vi "Test HP3488A.vi"() -> ()   [LabVIEW 2015]
panel:
  in  "Card Number":u8=1 min=1 max=5 step=1
  in  "VISA resource name":refnum<visa-resource-name>
  in  "stop":bool
  in  "Channel to select":T1(ring)
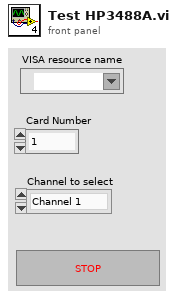
[diagram p1: front panel]
types:
  T1 = enum16{"Channel 1", "Channel 2", "Channel 3", "Channel 4"}
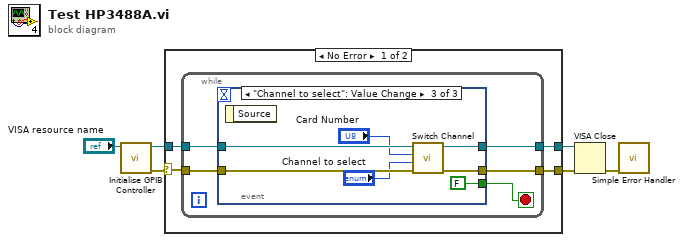
[diagram p0: block diagram]
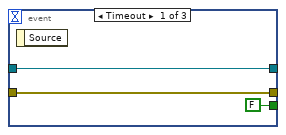
[diagram p2: hidden frame]
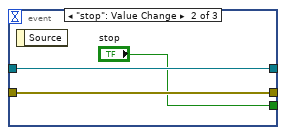
[diagram p3: hidden frame]
diagram:
  n1 = call "Initialise GPIB Controller.vi"("VISA resource name"="VISA resource name") -> ("error out"=w2:errorcluster, "VISA resource name out"=w6:refnum<visa-resource-name>)  [unwired: 5 in]
  n2 = case shown="No Error" w2 {
    selector: w2 -> [w7 w29]
    tunnel: w6 -> [w10 w30]
    tunnel: [w9 w30] -> w5
    tunnel: [w8 w29] -> w4
    frame No Error {
      n3 = while {
        tunnel: w10 -> [w15]
        tunnel: w7 -> [w14]
        tunnel: [w13] -> w9
        tunnel: [w12] -> w8
        stop <- w11 stop-if-true
        n4 = event shown="[2] \"Channel to select\": Value Change" {
          selector: _ -> [_ _ _]
          dyn-events: _ -> [_ _ _]
          timeout: _ -> [_ _ _]
          tunnel: w15 -> [w18 w21 w28]
          tunnel: w14 -> [w17 w20 w27]
          tunnel: [w18 w21 w26] -> w13
          tunnel: [w17 w20 w25] -> w12
          tunnel: [FALSE "stop" FALSE] -> w11
          event Timeout {
            n5 = event-data() -> ()  [unwired: 1 in, 1 out]
          }
          event "stop": Value Change {
            n6 = event-data() -> ()  [unwired: 1 in, 1 out]
          }
          event "Channel to select": Value Change {
            n7 = event-data() -> ()  [unwired: 1 in, 1 out]
            n8 = call "Switch Channel.vi"("error in (no error)"=w27, "Channel to select"="Channel to select", "Card Number"="Card Number", "VISA resource in"=w28) -> ("error out"=w25:errorcluster, "VISA resource out"=w26:refnum<visa-resource-name>)  [unwired: 2 in]
          }
        }
      }
    }
    frame Error {
    }
  }
  n9 = VISA Close(VISA resource name=w5, error in (no error)=w4) -> (error out=w1:errorcluster)
  n10 = call <vilib>:"Simple Error Handler.vi"("error in (no error)"=w1) -> ()  [unwired: 4 in, 5 out]
